vi "Format Dialog.vi"(0 "error handler in":refnum<class "TLB` Error Handler.lvclass">, 11 "error in":errorcluster) -> (4 "error handler out":refnum<class "TLB` Error Handler.lvclass">, 6 "source text":string, 15 "error out":errorcluster)   [LabVIEW 2023, in "TLB` InstStu GPlugin Template.lvlib" / "TLB` Error Handler.lvclass"]
uses:
  TLB` Error Handler.lvclass
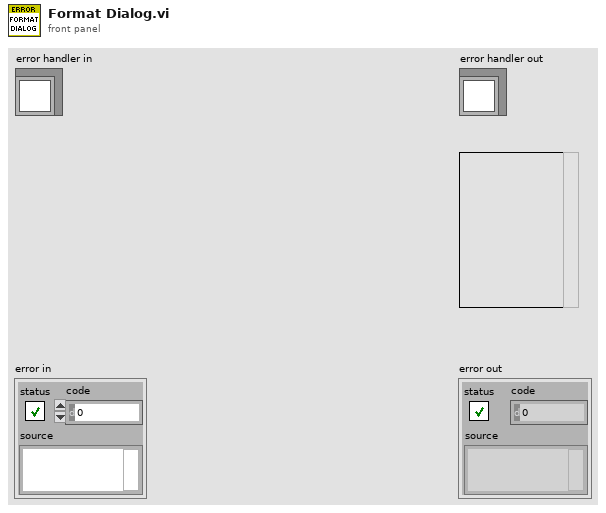
[diagram p1: front panel]
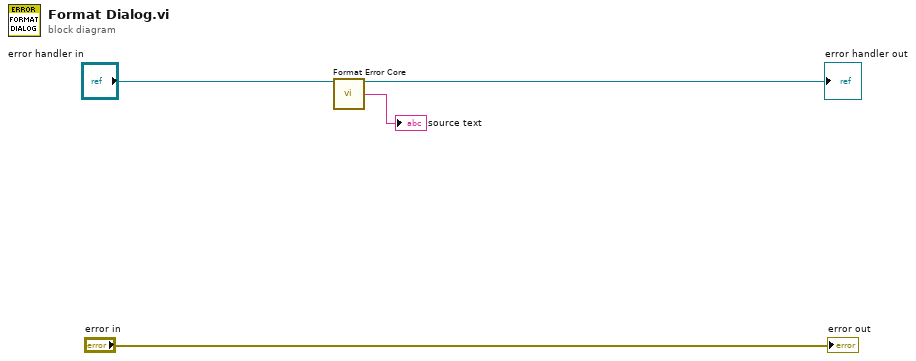
[diagram p0: block diagram]
diagram:
  n1 = call "Format Error Core.vi"("error handler in"="error handler in") -> ("error handler out"=→"error handler out":refnum<class "TLB` Error Handler.lvclass">, "source text"=→"source text":string)  [unwired: 13 in]
  "error out" <- "error in"
